vi "JSONconfig_RFSource.vi"(2 "error in (no error)":errorcluster, 3 "String":string, 4 "RF Block Input Array in":T1[](array[typedef])) -> (0 "error out":errorcluster, 1 "RF Block Input Array out":T1[](array[typedef]))   [LabVIEW 2019]
uses:
  Controls/RFBlockControl.ctl
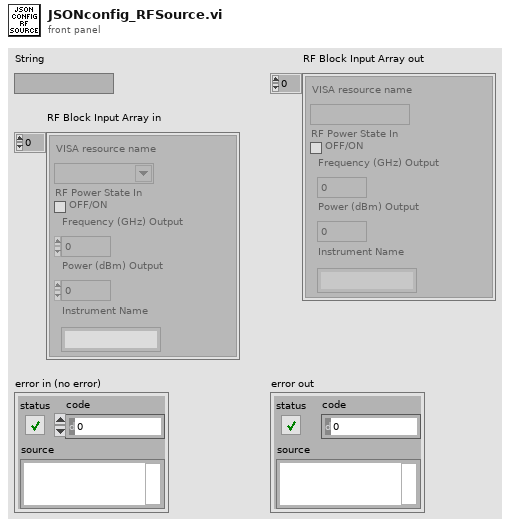
[diagram p1: front panel]
types:
  T1 = typedef "RFBlockControl.ctl" = cluster{"VISA resource name":refnum<visa-resource-name>, "RF Power State In":bool, "Frequency (GHz) Output":dbl, "Power (dBm) Output":dbl, "Instrument Name":string}
  T2 = cluster{"Gen_Array":cluster{"GPIB_address":dbl, "signal_name":string, "frequency":dbl, "power":dbl}[], "Gen_Number":dbl}
  T3 = cluster{"GPIB_address":dbl, "signal_name":string, "frequency":dbl, "power":dbl}[]
  T4 = cluster{"VISA resource name out":refnum<visa-resource-name>, bool, dbl, "power":dbl, "signal_name":string}
  T5 = cluster{"VISA resource name":refnum<visa-resource-name>, bool, "power":dbl, dbl, "signal_name":string}
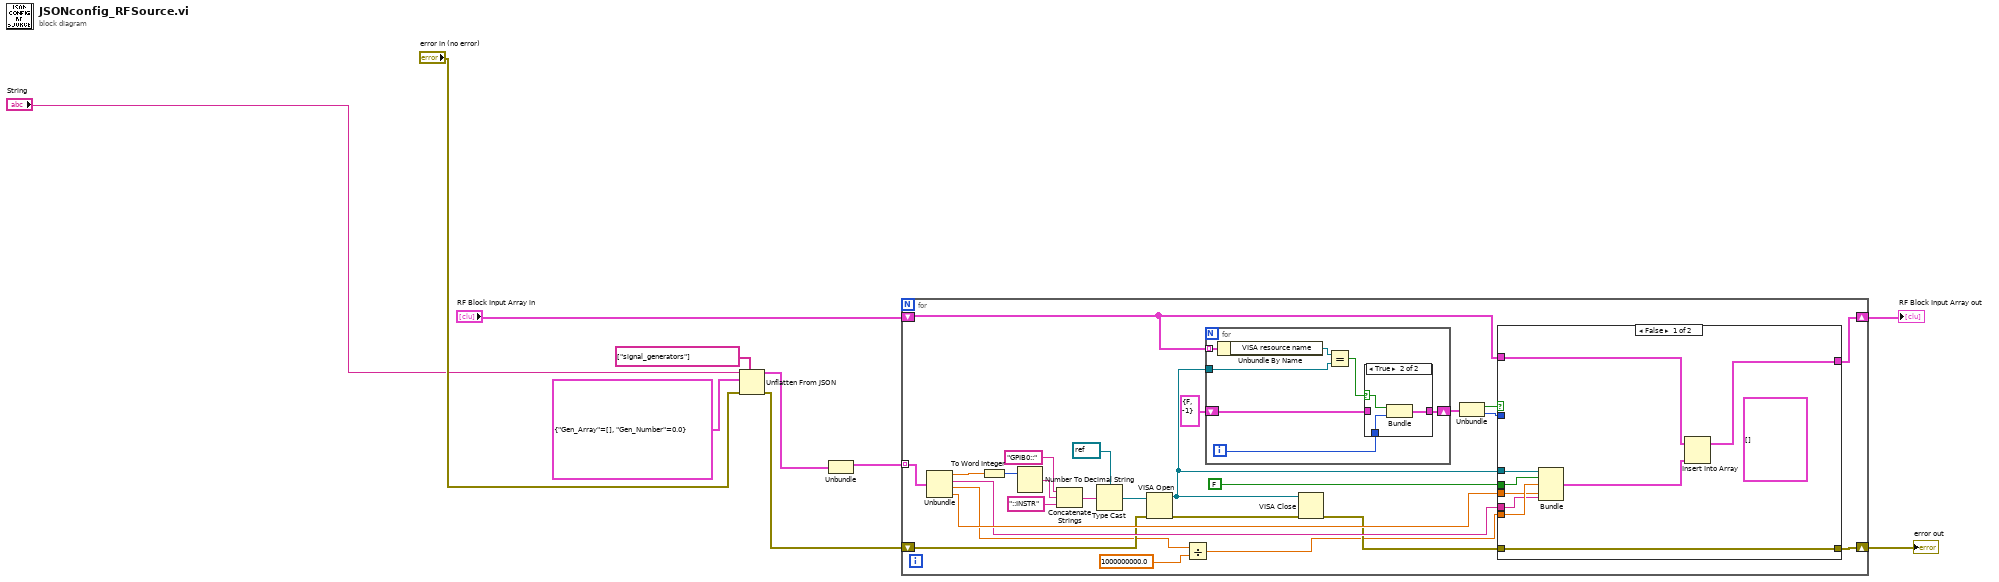
[diagram p0: block diagram]
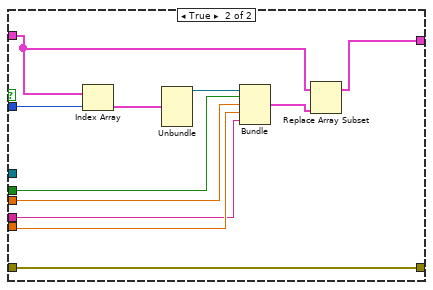
[diagram p2: hidden frame]
diagram:
  n1 = Unflatten From JSON(path=string[] ["signal_generators"], JSON string="String", type and defaults=T2 {"Gen_Array"=[], "Gen_Number"=0.0} ("cluster"), error in (no error)="error in (no error)") -> (value=w5:T2, error out=w7:errorcluster)  [unwired: 3 in]
  n2 = Unbundle(w5) -> ("Gen_Array"=w6:T3)  [unwired: 1 out]
  n3 = for {
    tunnel: w6 -> [w36] mode=indexing
    shift-right: [w24] -> w9
    shift-left: w7 -> [w23]
    shift-right: [w26] -> w10
    shift-left: "RF Block Input Array in" -> [w27]
    n4 = Unbundle(w36) -> ("GPIB_address"=w20:dbl, "signal_name"=w28:string, "frequency"=w12:dbl, "power"=w29:dbl)
    n5 = To Word Integer(number=w20) -> (16bit integer=w19:i16)
    n6 = Number To Decimal String(number=w19) -> (decimal integer string=w21:string)  [unwired: 1 in]
    n7 = Concatenate Strings("GPIB0::" ("string"), w21, "::INSTR" ("string")) -> (w17:string)
    n8 = Type Cast(type=refnum<visa-resource-name> refnum ("VISA resource name out"), x=w17) -> (*(type *) &x=w16:refnum<visa-resource-name>)
    n9 = VISA Open(error in (no error)=w23, VISA resource name=w16) -> (VISA resource name=w15:refnum<visa-resource-name>, error out=w14:errorcluster)  [unwired: 3 in]
    n10 = Divide(x=w12, y=1000000000.0) -> (x/y=w11:dbl)
    n11 = for {
      tunnel: w27 -> [w63] mode=indexing
      tunnel: w15 -> [w61]
      shift-right: [w58] -> w32
      shift-left: cluster{bool, i32} {FALSE, -1} -> [w59]
      i -> [w57]
      n12 = Unbundle By Name(w63) -> ("VISA resource name"=w62:refnum<visa-resource-name>)
      n13 = Equal?(x=w62, y=w61) -> (x = y?=w60:bool)
      n14 = case shown="True" w60 {
        selector: w60 -> [_ w66]
        tunnel: w59 -> [w64 _]
        tunnel: [w64 w67] -> w58
        tunnel: w57 -> [_ w65]
        frame False {
        }
        frame True {
          n15 = Bundle(w66, w65) -> (w67:cluster{bool, i32})  [unwired: 1 in]
        }
      }
    }
    n16 = VISA Close(VISA resource name=w15, error in (no error)=w14) -> (error out=w22:errorcluster)
    n17 = Unbundle(w32) -> (w31:bool, w25:i32)
    n18 = case shown="False" w31 {
      tunnel: w15 -> [w45 _]
      tunnel: FALSE -> [w44 w53]
      tunnel: w11 -> [w43 w51]
      tunnel: w29 -> [w42 w52]
      tunnel: w28 -> [w41 w50]
      tunnel: w27 -> [w39 w49]
      tunnel: [w38 w47] -> w26
      tunnel: w25 -> [_ w56]
      tunnel: [w37 w46] -> w24
      tunnel: w22 -> [w37 w46]
      frame False {
        (unwired) T1[] [] ("RF Block Input Array")
        n19 = Bundle("VISA resource name out"=w45, w44, w43, "power"=w42, "signal_name"=w41) -> (w40:T4)  [unwired: 1 in]
        n20 = Insert Into Array(array=w39, new element=w40) -> (w38:T1[])  [unwired: 1 in]
      }
      frame True {
        n21 = Index Array(array=w49, index=w56) -> (element=w55:T1)
        n22 = Unbundle(w55) -> ("VISA resource name"=w54:refnum<visa-resource-name>)  [unwired: 4 out]
        n23 = Bundle("VISA resource name"=w54, w53, "power"=w52, w51, "signal_name"=w50) -> (w48:T5)  [unwired: 1 in]
        n24 = Replace Array Subset(array=w49, new element=w48) -> (w47:T1[])  [unwired: 1 in]
      }
    }
  }
  "RF Block Input Array out" <- w10
  "error out" <- w9
